vi "Inst.Krohn-Hite-7008.InitSimChannels.vi"(11 "allChannelProperties":T1 {"channel" min=1 max=8 step=1}) -> (3 "allChannelProperties":T1 {"channel" min=1 max=8 step=1})   [LabVIEW 2019, in "Inst.KH7008.lvlib" / "Inst.Krohn-Hite-7008.lvclass"]
uses:
  Inst.Krohn-Hite-7008.lvclass
  KH7008/typedefs/allChannelProperties--Array.ctl
  KH7008/typedefs/channelProperties--Cluster.ctl
  KH7008/typedefs/channel--numeric.ctl
  KH7008/typedefs/gain--enum.ctl
  KH7008/typedefs/Input--Enum.ctl
  KH7008/typedefs/shunt--enum.ctl
  KH7008/typedefs/couple--Enum.ctl
  KH7008/typedefs/Filter--Enum.ctl
  <vilib>/numeric/Random Number (Range) U64.vi
  <vilib>/numeric/sub_Random U32.vi
  KH7008/KH7008.lvlib
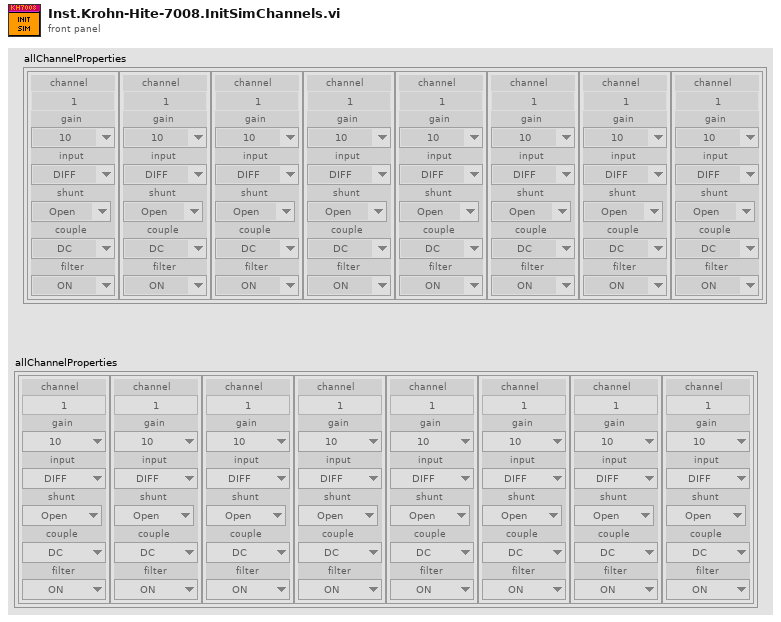
[diagram p1: front panel]
types:
  T1 = typedef "KH7008.lvlib/allChannelProperties--Array.ctl" = T2[]
  T2 = typedef "KH7008.lvlib/channelProperties--Cluster.ctl" = cluster{"channel":T3, "gain":T4, "input":T5, "shunt":T6, "couple":T7, "filter":T8}
  T3 = typedef "KH7008.lvlib/channel--numeric.ctl" = u16
  T4 = typedef "KH7008.lvlib/gain--enum.ctl" = enum16{"1", "10", "100", "1000"}
  T5 = typedef "KH7008.lvlib/input--enum.ctl" = enum16{"OFF", "SE+", "SE-", "DIFF"}
  T6 = typedef "KH7008.lvlib/shunt--enum.ctl" = enum16{"Open", "50", "500", "5k", "50k", "10M"}
  T7 = typedef "KH7008.lvlib/couple--enum.ctl" = enum16{"AC", "DC"}
  T8 = typedef "KH7008.lvlib/filter--enum.ctl" = enum16{"OFF", "ON"}
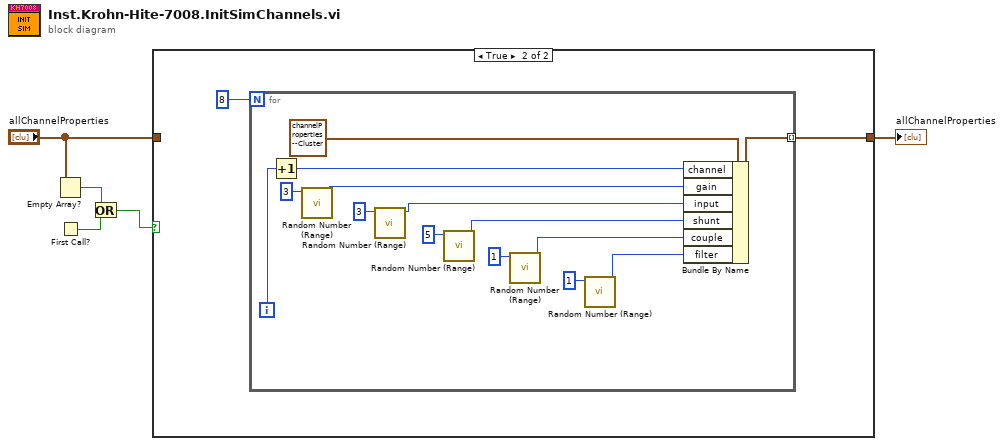
[diagram p0: block diagram]
diagram:
  n1 = Empty Array?(array="allChannelProperties") -> (empty?=w5:bool)
  n2 = First Call?() -> (First Call?: T/F=w4:bool)
  n3 = Or(x=w5, y=w4) -> (x .or. y?=w3:bool)
  n4 = case shown="True" w3 {
    tunnel: [w6 w7] -> w2
    tunnel: "allChannelProperties" -> [w6 _]
    frame False {
    }
    frame True {
      n5 = for {
        N: 8 -> [_]
        tunnel: [w21] -> w7 mode=indexing
        i -> [w19]
        n6 = Increment(x=w19) -> (x+1=w20:i32)
        n7 = call-poly <vilib>:"Random Number (Range).vi"("upper bound (100)"=u64 3) -> ("number"=w13:u64)  [unwired: 10 in]
        n8 = call-poly <vilib>:"Random Number (Range).vi"("upper bound (100)"=u64 3) -> ("number"=w12:u64)  [unwired: 10 in]
        n9 = call-poly <vilib>:"Random Number (Range).vi"("upper bound (100)"=u64 5) -> ("number"=w11:u64)  [unwired: 10 in]
        n10 = call-poly <vilib>:"Random Number (Range).vi"("upper bound (100)"=u64 1) -> ("number"=w10:u64)  [unwired: 10 in]
        n11 = call-poly <vilib>:"Random Number (Range).vi"("upper bound (100)"=u64 1) -> ("number"=w9:u64)  [unwired: 10 in]
        n12 = Bundle By Name(cluster=T2 {"channel"=1, "gain"=enum."10", "input"=enum."DIFF", "shunt"=enum."Open", "couple"=enum."DC", "filter"=enum."ON"} ("channelProperties"), "channel"=w20, "gain"=w13, "input"=w12, "shunt"=w11, "couple"=w10, "filter"=w9) -> (w21:T2)
      }
    }
  }
  "allChannelProperties" <- w2
